vi "PmacCoordMotorToEncoder.vi"(2 "Input Value Double":dbl format="%.2f", 3 "Coord Specify Cluster":T1 {"Coord Number i32 (1-8) (1)" min=1 max=8; "Motor Number i32 (1-8) (1)" min=1 max=8}, 4 "Device Number i32 (0)":i32 min=0) -> (0 "Output Value Double":dbl format="%.2f", 1 "Coord Defined Bool":bool)   [LabVIEW 2020]
doc: "Coord Specify Cluster specifies a motor within a CS and an attempt to convert Input Value from CS units to encoder counts. If the motor is not defined in the CS no conversions is applied. If the motor is defined and Convert is TRUE Coord Defined is TRUE and Output Value is scaled from CS units to encoder counts."
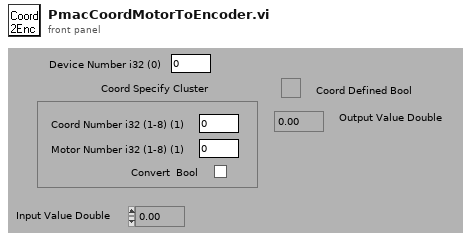
[diagram p1: front panel]
types:
  T1 = cluster{"Coord Number i32 (1-8) (1)":i32, "Motor Number i32 (1-8) (1)":i32, "Convert  Bool":bool}
  T2 = cluster{"Definition String":string[], "Scale Factor":i32[], "Defined":bool[], "Coordinate System":i32}
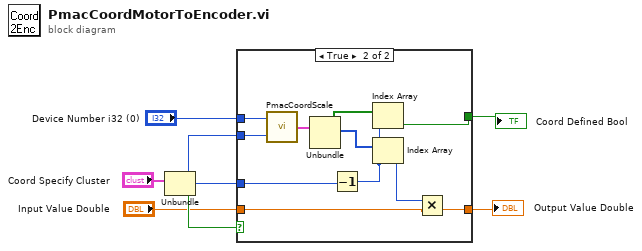
[diagram p0: block diagram]
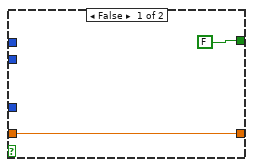
[diagram p2: hidden frame]
diagram:
  n1 = Unbundle("Coord Specify Cluster") -> ("Coord Number i32 (1-8) (1)"=w4:i32, "Motor Number i32 (1-8) (1)"=w3:i32, "Convert  Bool"=w6:bool)
  n2 = case shown="True" w6 {
    tunnel: [FALSE w19] -> w7
    tunnel: "Device Number i32 (0)" -> [_ w16]
    tunnel: w4 -> [_ w15]
    tunnel: w3 -> [_ w14]
    tunnel: "Input Value Double" -> [w9 w12]
    tunnel: [w9 w11] -> w1
    frame False {
    }
    frame True {
      n3 = call "PmacCoordScale.vi"("Coord Number i32 (1-8) (1)"=w15, "Device Number i32 (0)"=w16) -> ("Coordinate System Scale Cluster"=w21:T2)
      n4 = Unbundle(w21) -> ("Scale Factor"=w18:i32[], "Defined"=w20:bool[])  [unwired: 2 out]
      n5 = Decrement(x=w14) -> (x-1=w17:i32)
      n6 = Index Array(array=w20, index=w17) -> (element=w19:bool)
      n7 = Index Array(array=w18, index=w17) -> (element=w13:i32)
      n8 = Multiply(x=w13, y=w12) -> (x*y=w11:dbl)
    }
  }
  "Output Value Double" <- w1
  "Coord Defined Bool" <- w7
